vi "Read Controls from Config File.vi"(6 "Child?":bool, 7 "section":string, 8 "Error In":errorcluster, 9 "ParentName":string, 10 "Ctl Refnum":refnum<vi>, 11 "refnum":T1) -> (0 "Error Out":errorcluster, 3 "refnum out":T1)   [LabVIEW 2018]
uses:
  <vilib>/Utility/config.llb/Config Data RefNum.ctl
  Hardware Mfg/Thorlabs Translation Stages/Controls/Translation Stage Cluster.ctl
  Controls/Translation Stage Types.ctl
  <vilib>/Utility/config.llb/Read Key (String).vi
  <vilib>/Utility/config.llb/Read Key (Boolean).vi
  <vilib>/Utility/config.llb/Read Key (Double).vi
  <vilib>/Utility/config.llb/Read Key (U32).vi
  <vilib>/Utility/config.llb/NI_LVConfig.lvlib
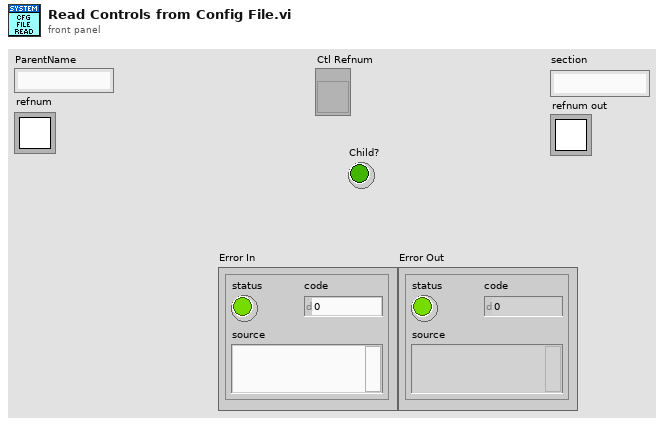
[diagram p1: front panel]
types:
  T1 = typedef "NI_LVConfig.lvlib/Config Data RefNum.ctl" = refnum<k1>
  T2 = typedef "Translation Stage Cluster.ctl" = cluster{"Position":dbl, "Is.Enabled?":bool, "Is.Connected?":bool, "Device SN":string, "AccelerationMaximum":dbl, "VelocityMaximum":dbl, "Acceleration":dbl, "Velocity":dbl, "waitTimeout (ms)":i32, "Model":T3, "Is.Homed?":bool}
  T3 = typedef "Translation Stage Types.ctl" = enum16{"None", "Thorlabs LTS", "Thorlabs MLJ"}
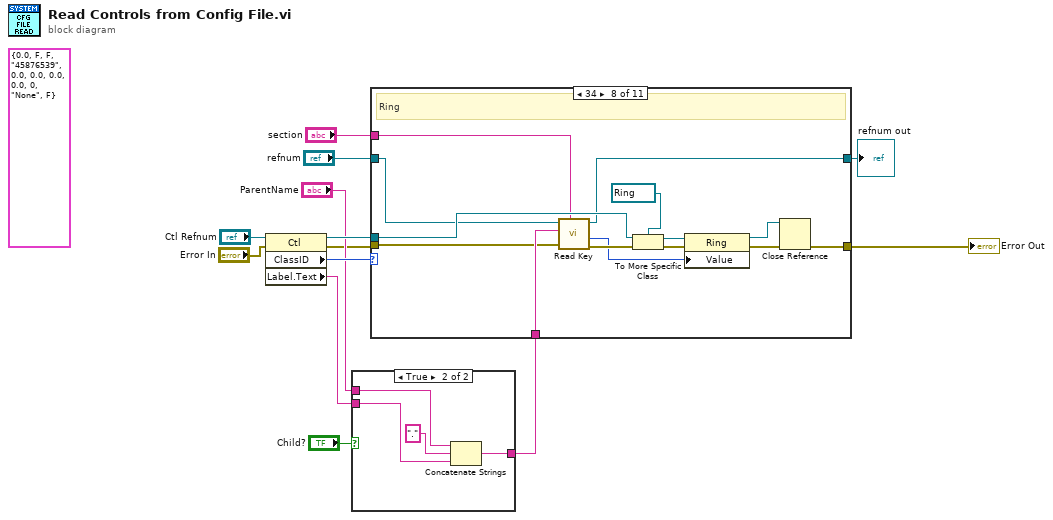
[diagram p0: block diagram]
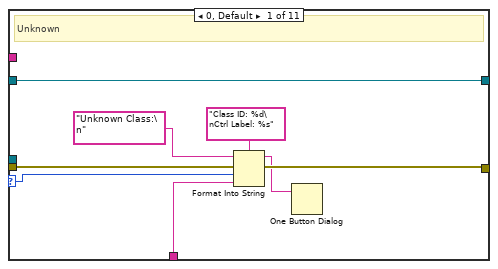
[diagram p3: hidden frame]
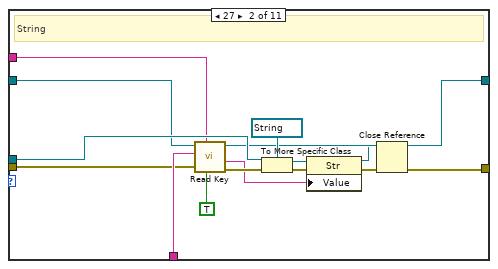
[diagram p4: hidden frame]
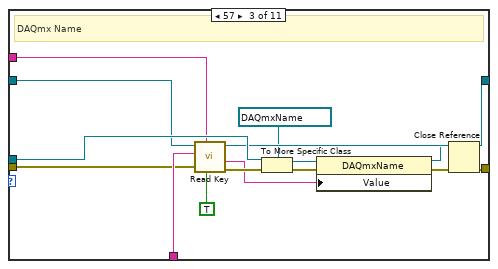
[diagram p5: hidden frame]
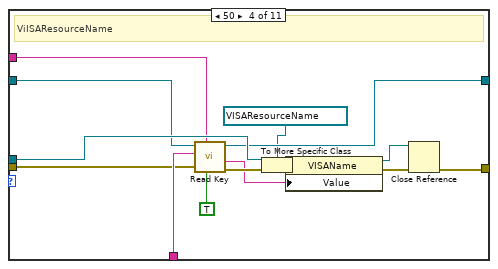
[diagram p6: hidden frame]
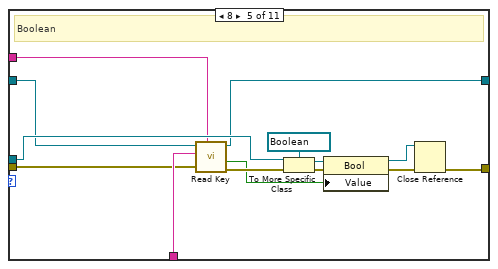
[diagram p7: hidden frame]
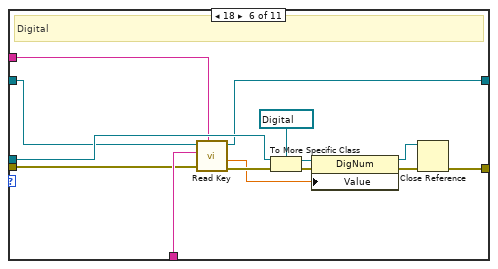
[diagram p8: hidden frame]
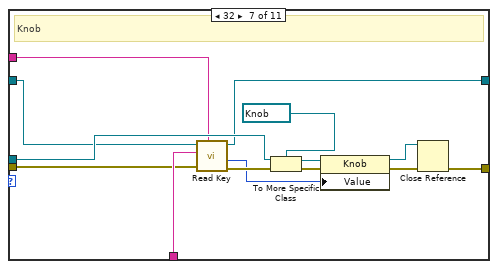
[diagram p9: hidden frame]
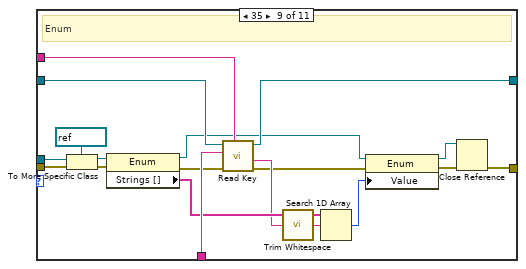
[diagram p10: hidden frame]
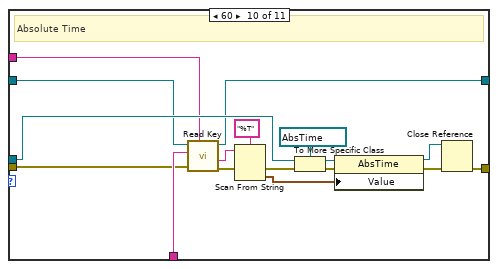
[diagram p11: hidden frame]
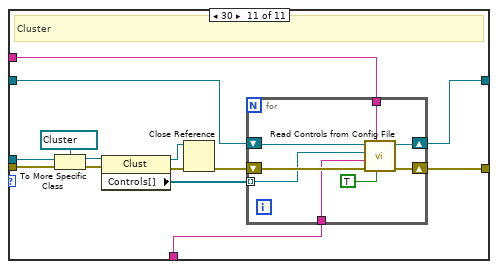
[diagram p12: hidden frame]
diagram:
  (unwired) T2 {"Position"=0.0, "Is.Enabled?"=FALSE, "Is.Connected?"=FALSE, "Device SN"="45876539", "AccelerationMaximum"=0.0, "VelocityMaximum"=0.0, "Acceleration"=0.0, "Velocity"=0.0, "waitTimeout (ms)"=0, "Model"=enum."None", "Is.Homed?"=FALSE} ("Control Param In")
  n1 = property class="Ctl"(reference="Ctl Refnum", error in="Error In") -> (reference out=w12:refnum<vi>, error out=w6:errorcluster, "ClassID"=w11:u32, "Label.Text"=w8:string)
  n2 = case shown="True" "Child?" {
    tunnel: "ParentName" -> [_ w18]
    tunnel: w8 -> [w14 w16]
    tunnel: [w14 w15] -> w3
    frame False {
    }
    frame True {
      n3 = Concatenate Strings(w18, ".", w16) -> (w15:string)
    }
  }
  n4 = case shown="34" w11 {
    selector: w11 -> [w23 _ _ _ _ _ _ _ _ _ _]
    tunnel: w6 -> [w21 w30 w46 w61 w73 w87 w102 w116 w145 w151 w176]
    tunnel: w12 -> [_ w40 w56 w71 w83 w98 w112 w126 w144 w162 w174]
    tunnel: [w20 w28 w44 w59 w82 w88 w103 w117 w128 w152 w170] -> w1
    tunnel: "section" -> [_ w39 w55 w70 w81 w91 w106 w120 w140 w156 w167]
    tunnel: "refnum" -> [w26 w38 w54 w69 w80 w90 w105 w119 w139 w155 w169]
    tunnel: [w26 w37 w53 w68 w79 w89 w104 w118 w138 w154 w168] -> w2
    tunnel: w3 -> [w22 w35 w51 w66 w77 w92 w107 w121 w141 w157 w166]
    frame 0, Default {
      # "Unknown"
      n5 = Format Into String(format string="Class ID: %d\nCtrl Label: %s", initial string="Unknown Class:\n" ("string"), error in=w21, w23, w22) -> (resulting string=w19:string, error out=w20:errorcluster)
      n6 = One Button Dialog(message=w19) -> ()  [unwired: 1 in, 1 out]
    }
    frame 27 {
      # "String"
      n7 = call-poly <vilib>:"Read Key.vi"("read raw string? (F)"=TRUE, "section"=w39, "error in (no error)"=w30, "key"=w35, "refnum"=w38) -> ("error out"=w29:errorcluster, "value"=w27:string, "refnum out"=w37:T1)  [unwired: 3 in, 1 out]
      n8 = To More Specific Class(target class=refnum<vi> refnum ("AccelerationMaximum 2"), reference=w40, error in=w29) -> (specific class reference=w33:refnum<vi>, error out=w36:errorcluster)
      n9 = property class="Str"(reference=w33, error in=w36, "Value"=w27) -> (reference out=w32:refnum<vi>, error out=w34:errorcluster)
      n10 = Close Reference(reference=w32, error in (no error)=w34) -> (error out=w28:errorcluster)
    }
    frame 57 {
      # "DAQmx Name"
      n11 = call-poly <vilib>:"Read Key.vi"("read raw string? (F)"=TRUE, "section"=w55, "error in (no error)"=w46, "key"=w51, "refnum"=w54) -> ("error out"=w45:errorcluster, "value"=w43:string, "refnum out"=w53:T1)  [unwired: 3 in, 1 out]
      n12 = To More Specific Class(target class=refnum<vi> refnum ("Analog Out Channel"), reference=w56, error in=w45) -> (specific class reference=w49:refnum<vi>, error out=w52:errorcluster)
      n13 = property class="DAQmxName"(reference=w49, error in=w52, "Value"=w43) -> (reference out=w48:refnum<vi>, error out=w50:errorcluster)
      n14 = Close Reference(reference=w48, error in (no error)=w50) -> (error out=w44:errorcluster)
    }
    frame 50 {
      # "ViISAResourceName"
      n15 = call-poly <vilib>:"Read Key.vi"("read raw string? (F)"=TRUE, "section"=w70, "error in (no error)"=w61, "key"=w66, "refnum"=w69) -> ("error out"=w60:errorcluster, "value"=w58:string, "refnum out"=w68:T1)  [unwired: 3 in, 1 out]
      n16 = To More Specific Class(target class=refnum<vi> refnum ("Controller VISA Ref"), reference=w71, error in=w60) -> (specific class reference=w64:refnum<vi>, error out=w67:errorcluster)
      n17 = property class="VISAName"(reference=w64, error in=w67, "Value"=w58) -> (reference out=w63:refnum<vi>, error out=w65:errorcluster)
      n18 = Close Reference(reference=w63, error in (no error)=w65) -> (error out=w59:errorcluster)
    }
    frame 8 {
      # "Boolean"
      n19 = call-poly <vilib>:"Read Key.vi"("section"=w81, "error in (no error)"=w73, "key"=w77, "refnum"=w80) -> ("error out"=w82:errorcluster, "value"=w72:bool, "refnum out"=w79:T1)  [unwired: 4 in, 1 out]
      n20 = To More Specific Class(target class=refnum<vi> refnum ("AccelerationMaximum 2"), reference=w83) -> (specific class reference=w75:refnum<vi>, error out=w78:errorcluster)  [unwired: 1 in]
      n21 = property class="Bool"(reference=w75, error in=w78, "Value"=w72) -> (reference out=w74:refnum<vi>, error out=w76:errorcluster)
      n22 = Close Reference(reference=w74, error in (no error)=w76) -> ()  [unwired: 1 out]
    }
    frame 18 {
      # "Digital"
      n23 = call-poly <vilib>:"Read Key.vi"("section"=w91, "error in (no error)"=w87, "key"=w92, "refnum"=w90) -> ("error out"=w86:errorcluster, "value"=w85:dbl, "refnum out"=w89:T1)  [unwired: 4 in, 1 out]
      n24 = To More Specific Class(target class=refnum<vi> refnum ("AccelerationMaximum 2"), reference=w98, error in=w86) -> (specific class reference=w95:refnum<vi>, error out=w96:errorcluster)
      n25 = property class="DigNum"(reference=w95, error in=w96, "Value"=w85) -> (reference out=w93:refnum<vi>, error out=w94:errorcluster)
      n26 = Close Reference(reference=w93, error in (no error)=w94) -> (error out=w88:errorcluster)
    }
    frame 32 {
      # "Knob"
      n27 = call-poly <vilib>:"Read Key.vi"("section"=w106, "error in (no error)"=w102, "key"=w107, "refnum"=w105) -> ("error out"=w101:errorcluster, "value"=w100:u32, "refnum out"=w104:T1)  [unwired: 4 in, 1 out]
      n28 = To More Specific Class(target class=refnum<vi> refnum ("Zoom Factor"), reference=w112, error in=w101) -> (specific class reference=w110:refnum<vi>, error out=w111:errorcluster)
      n29 = property class="Knob"(reference=w110, error in=w111, "Value"=w100) -> (reference out=w108:refnum<vi>, error out=w109:errorcluster)
      n30 = Close Reference(reference=w108, error in (no error)=w109) -> (error out=w103:errorcluster)
    }
    frame 34 {
      # "Ring"
      n31 = call-poly <vilib>:"Read Key.vi"("section"=w120, "error in (no error)"=w116, "key"=w121, "refnum"=w119) -> ("error out"=w115:errorcluster, "value"=w114:u32, "refnum out"=w118:T1)  [unwired: 4 in, 1 out]
      n32 = To More Specific Class(target class=refnum<vi> refnum ("Trigger Operation"), reference=w126, error in=w115) -> (specific class reference=w124:refnum<vi>, error out=w125:errorcluster)
      n33 = property class="Ring"(reference=w124, error in=w125, "Value"=w114) -> (reference out=w122:refnum<vi>, error out=w123:errorcluster)
      n34 = Close Reference(reference=w122, error in (no error)=w123) -> (error out=w117:errorcluster)
    }
    frame 35 {
      # "Enum"
      n35 = To More Specific Class(target class=refnum<vi> refnum ("Enum"), reference=w144, error in=w145) -> (specific class reference=w142:refnum<vi>, error out=w143:errorcluster)
      n36 = property class="Enum"(reference=w142, error in=w143) -> (reference out=w129:refnum<vi>, error out=w135:errorcluster, "Strings []"=w136:string[])
      n37 = call-poly <vilib>:"Read Key.vi"("section"=w140, "error in (no error)"=w135, "key"=w141, "refnum"=w139) -> ("error out"=w133:errorcluster, "value"=w134:string, "refnum out"=w138:T1)  [unwired: 4 in, 1 out]
      n38 = call <vilib>:"Trim Whitespace.vi"("string"=w134) -> ("trimmed string"=w131:string)  [unwired: 1 in]
      n39 = Search 1D Array(1D array=w136, element=w131) -> (index of element=w130:i32)  [unwired: 1 in]
      n40 = property class="Enum"(reference=w129, error in=w133, "Value"=w130) -> (reference out=w127:refnum<vi>, error out=w132:errorcluster)
      n41 = Close Reference(reference=w127, error in (no error)=w132) -> (error out=w128:errorcluster)
    }
    frame 60 {
      # "Absolute Time"
      n42 = call-poly <vilib>:"Read Key.vi"("section"=w156, "error in (no error)"=w151, "key"=w157, "refnum"=w155) -> ("error out"=w149:errorcluster, "value"=w146:string, "refnum out"=w154:T1)  [unwired: 4 in, 1 out]
      n43 = Scan From String(format string="%T", input string=w146, error in=w149) -> (error out=w148:errorcluster, output 1=w147:timestamp)  [unwired: 2 in, 2 out]
      n44 = To More Specific Class(target class=refnum<vi> refnum ("AccelerationMaximum 2"), reference=w162, error in=w148) -> (specific class reference=w160:refnum<vi>, error out=w161:errorcluster)
      n45 = property class="AbsTime"(reference=w160, error in=w161, "Value"=w147) -> (reference out=w158:refnum<vi>, error out=w159:errorcluster)
      n46 = Close Reference(reference=w158, error in (no error)=w159) -> (error out=w152:errorcluster)
    }
    frame 30 {
      # "Cluster"
      n47 = To More Specific Class(target class=refnum<vi> refnum ("Cluster Ref In"), reference=w174, error in=w176) -> (specific class reference=w172:refnum<vi>, error out=w173:errorcluster)
      n48 = property class="Clust"(reference=w172, error in=w173) -> (reference out=w164:refnum<vi>, error out=w171:errorcluster, "Controls[]"=w163:refnum<vi>[])
      n49 = Close Reference(reference=w164, error in (no error)=w171) -> (error out=w165:errorcluster)
      n50 = for {
        tunnel: w167 -> [w180]
        tunnel: w166 -> [w179]
        shift-right: [w183] -> w170
        shift-left: w165 -> [w184]
        shift-right: [w181] -> w168
        shift-left: w169 -> [w182]
        tunnel: w163 -> [w177] mode=indexing
        n51 = call "Read Controls from Config File.vi"("Child?"=TRUE, "section"=w180, "Error In"=w184, "ParentName"=w179, "Ctl Refnum"=w177, "refnum"=w182) -> ("Error Out"=w183:errorcluster, "refnum out"=w181:T1)  [unwired: 4 in]
      }
    }
  }
  "Error Out" <- w1
  "refnum out" <- w2
